vi "CRYConfigure Step.vi"(11 "Project Tree reference":refnum<vi>) -> (1 "Steps config.":bool[](array[boolean]))   [LabVIEW 2013]
uses:
  <vilib>/Utility/miscctls.llb/LVStringsAndValuesArrayTypeDef.ctl
  CRYProject Editor Global.vi
panel:
  in  "Unit":string caption="单位"
  in  "Comment":string caption="注解"
  in  "Name":string caption="名字"
  in  "Overwrite":u16(slide) caption="UseMLVal_Level_1"
  in  "Y unit":string
  in  "Y dB ref":dbl=1.0 format="%.1f"
  in  "Y prefix":string
  in  "Y data":u16(ring)=1 items=["dB", "Lin"]
  in  "btnUnit":bool caption="units"
  in  "Iterations":i32 caption="迭代"
  in  "Increment":dbl=1.0 caption="增量" min=1.0 step=1.0
  in  "Start":dbl caption="开始" format="%#_5g"
  in  "Load Test":bool
  in  "After":bool caption="后"
  in  "counts jump":i32(ring)=4 items=["激励"=1, "采集"=2, "分析"=3, "后处理"=4, "上下限"=5]
  in  "fail jump":i32(ring)=4 items=["激励"=1, "采集"=2, "分析"=3, "后处理"=4, "上下限"=5]
  in  "pass jump":i32(ring)=4 items=["激励"=1, "采集"=2, "分析"=3, "后处理"=4, "上下限"=5]
  in  "Jump on FAIL to":bool caption="失败时跳转"
  in  "Jump on PASS to":bool caption="通过时跳转"
  in  "Halt on PASS":bool caption="通过时停止"
  in  "Halt on FAIL":bool caption="失败时停止"
  in  "Default action for new steps":bool caption="默认动作为新步骤"
  out "Step Name":string
  in  "wait for confirmation?":bool caption="显示确认"
  in  "Cancel button":bool
  in  "OK button":bool
  # "..................."
  # "..................."
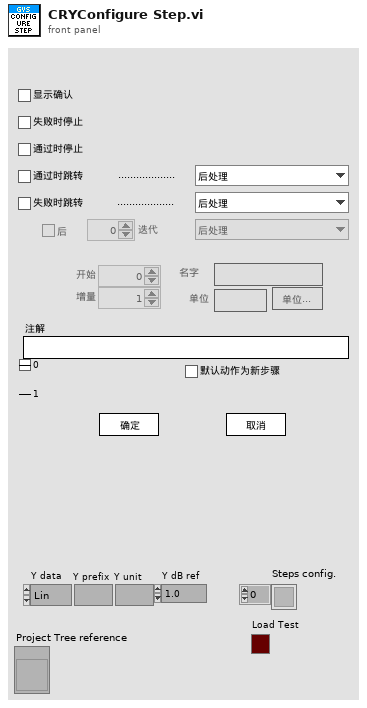
[diagram p1: front panel]
types:
  T1 = typedef "LVStringsAndValuesArrayTypeDef.ctl" = cluster{"String":string, "Value":ext}[]
  T2 = typedef "CRYTS.ctl" = cluster{"No.TS":u16, "TS File Path":path, "TS Name":string, "EditStepName":string, "Steps":T3[], "New State":bool, "Change State":bool, "Flattened CurveLib Data":string, "Document Data":string, "EditStepNo":u16, "Operator Start File":string, "Sequence Type":string, "Sequence Language":string}
  T3 = typedef "CRYStep.ctl" = cluster{"No.VI":i32, "Category":string, "StepName":string, "Seq setup flattened":string, "Comment":string, "Steps config.":bool[], "Jump config":i32[], "Start":dbl, "Increment":dbl, "Name":string, "Unit":string, "Y data":u16, "Y prefix":string, "Y dB ref":dbl, "Y unit":string, "Repeat State Array":cluster{"Start":dbl, "Increment":dbl, "Count":i32, "Num":i32}[]}
  T4 = typedef "CRYStart Cluster.ctl" = cluster{"SequenceName":string, "Preload Stimulus":bool, "CloseOpenedDisplay":bool, "ClearMeasuredData":bool, "UpdateDisplayDuringRun":bool, "DisplayForConfirmation":bool, "HaltOnFail":bool, "UseSameHardware":bool, "UseSameCalibration":bool}
  T5 = enum8{"Enabled", "Disabled", "Disabled and Grayed Out"}
  T6 = enum16{"Curves", "Values", "Results", "WFM", "All"}
  T7 = cluster{"SourceRowNum":i32, "SourceCount":i32, "TargetRowNum":i32, "bResult":bool, "EditRowNum":i32}
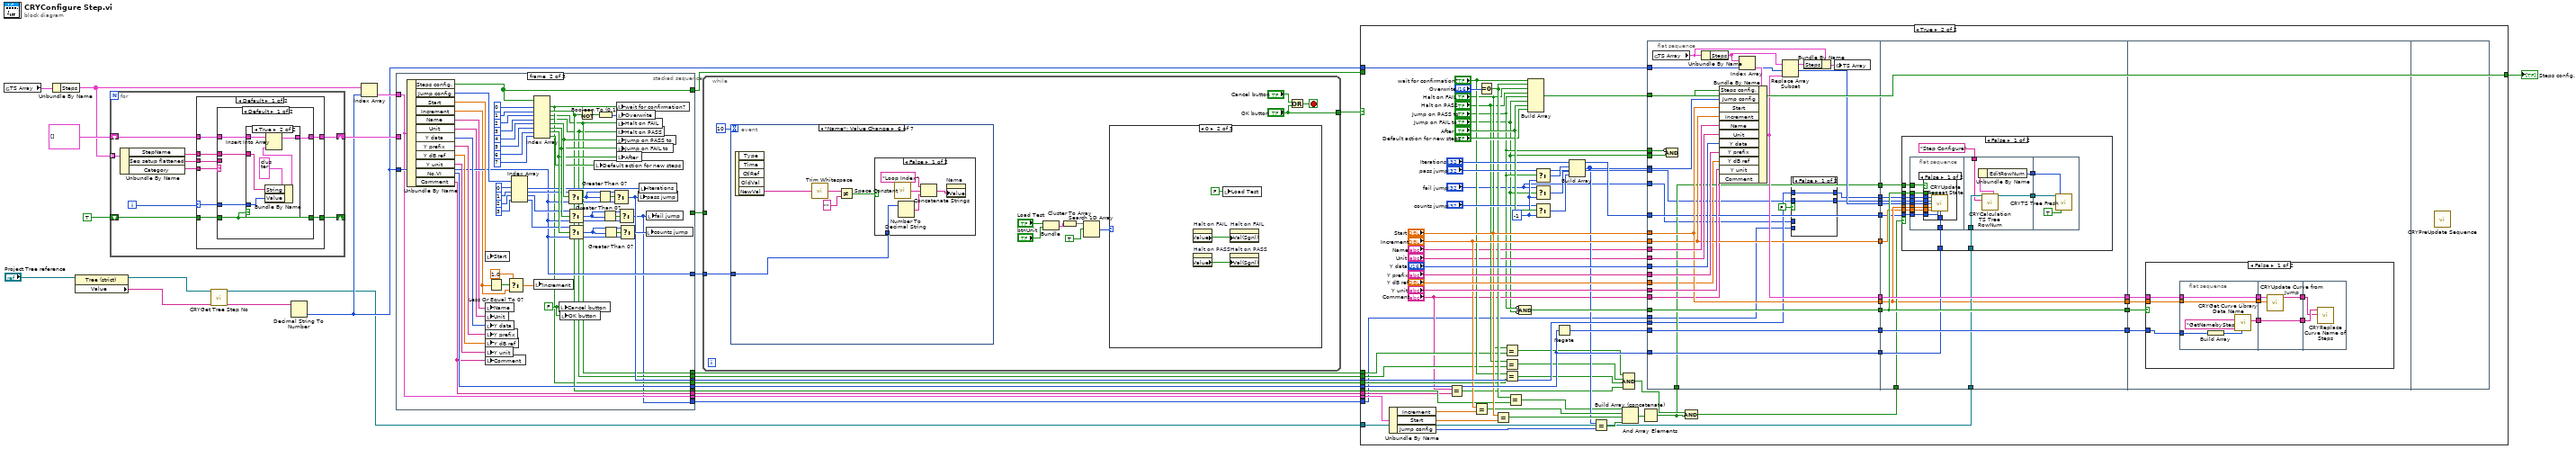
[diagram p0: block diagram]
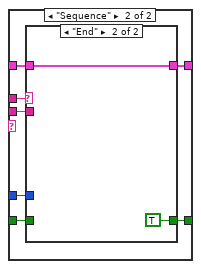
[diagram p3: hidden frame]
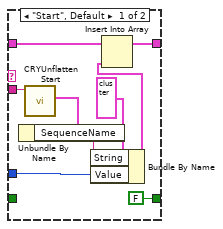
[diagram p4: hidden frame]
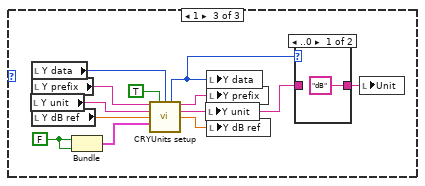
[diagram p7: hidden frame]
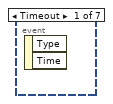
[diagram p9: hidden frame]
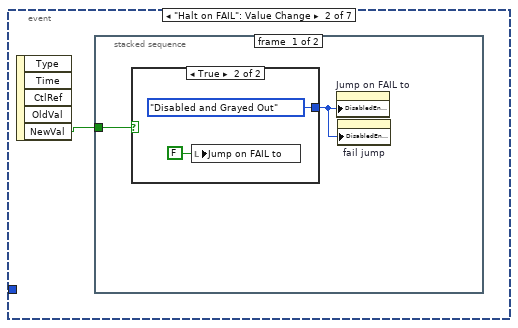
[diagram p10: hidden frame]
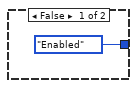
[diagram p11: hidden frame]
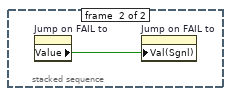
[diagram p12: hidden frame]
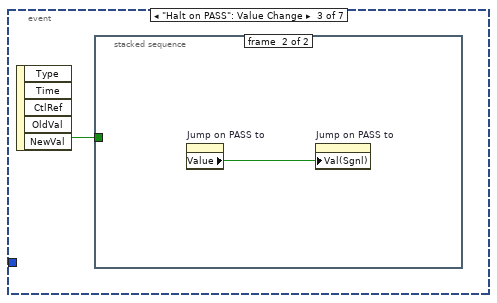
[diagram p13: hidden frame]
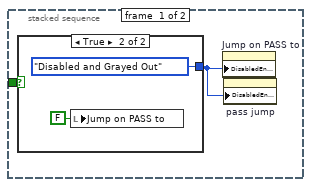
[diagram p14: hidden frame]
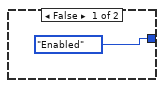
[diagram p15: hidden frame]
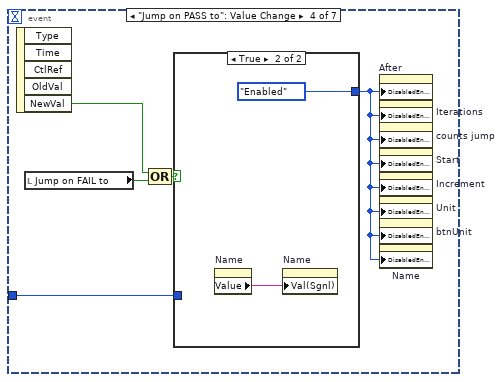
[diagram p16: hidden frame]
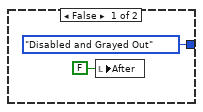
[diagram p17: hidden frame]
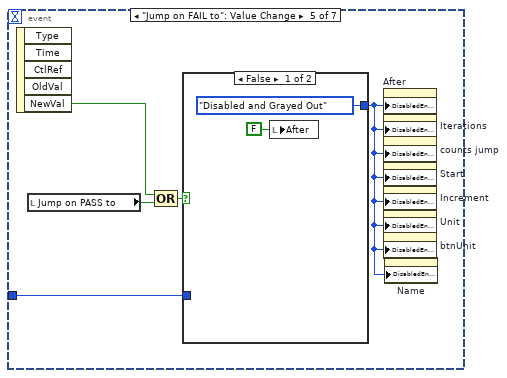
[diagram p18: hidden frame]
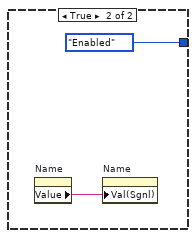
[diagram p19: hidden frame]
diagram:
  n1 = global read "CRYProject Editor Global.vi" "TS Array"() -> (w24:T2)
  n2 = Unbundle By Name(w24) -> ("Steps"=w16:T3[])
  n3 = property on="Property Node" class="Tree (strict)"(reference="Project Tree reference") -> (reference out=w7:refnum<vi>, "Value"=w6:string)  [unwired: 1 in, 1 out]
  n4 = for {
    tunnel: w16 -> [w34] mode=indexing
    shift-right: [w33] -> w18
    shift-left: T1 [] ("Strings And Values []") -> [w35]
    shift-right: [w30] -> _
    shift-left: TRUE ("Cancel button") -> [w31]
    i -> [w28]
    n5 = Unbundle By Name(w34) -> ("StepName"=w29:string, "Seq setup flattened"=w32:string, "Category"=w27:string)
    n6 = case shown="Default" w28 {
      selector: w28 -> [w39 _]
      tunnel: w35 -> [w42 w75]
      tunnel: [w40 w75] -> w33
      tunnel: w29 -> [w43 _]
      tunnel: w32 -> [w41 _]
      tunnel: w31 -> [w38 w74]
      tunnel: [w37 w74] -> w30
      tunnel: w27 -> [w36 _]
      frame Default {
        n7 = case shown="Default" w36 {
          tunnel: w43 -> [w45 w62]
          tunnel: w42 -> [w48 w61]
          tunnel: w41 -> [_ w60]
          tunnel: [w44 w59] -> w40
          tunnel: w39 -> [w46 w58]
          tunnel: w38 -> [w47 w57]
          tunnel: [w47 w56] -> w37
          frame Default {
            n8 = case shown="True" w47 {
              tunnel: w48 -> [w49 w55]
              tunnel: [w49 w54] -> w44
              tunnel: w45 -> [_ w52]
              tunnel: w46 -> [_ w51]
              frame False {
              }
              frame True {
                n9 = Bundle By Name(cluster=cluster{"String":string, "Value":ext} {"String"="", "Value"=0.0}, "String"=w52, "Value"=w51) -> (w50:cluster{"String":string, "Value":ext})
                n10 = Insert Into Array(array=w55, new element=w50) -> (w54:T1)  [unwired: 1 in]
              }
            }
          }
          frame "Sequence" {
            n11 = case shown="\"End\"" w62 {
              tunnel: w61 -> [w71 w73]
              tunnel: [w70 w73] -> w59
              tunnel: w60 -> [w69 _]
              tunnel: w58 -> [w64 _]
              tunnel: w57 -> [_ _]
              tunnel: [FALSE ("Cancel button") TRUE ("Cancel button")] -> w56
              frame "Start", Default {
                n12 = call "CRYUnflatten Start.vi"("Unflatten Sequence"=w69) -> ("Sequence Configure"=w68:T4)  [unwired: 8 in, 2 out]
                n13 = Unbundle By Name(w68) -> ("SequenceName"=w65:string)
                n14 = Bundle By Name(cluster=cluster{"String":string, "Value":ext} {"String"="", "Value"=0.0}, "String"=w65, "Value"=w64) -> (w63:cluster{"String":string, "Value":ext})
                n15 = Insert Into Array(array=w71, new element=w63) -> (w70:T1)  [unwired: 1 in]
              }
              frame "End" {
              }
            }
          }
        }
      }
      frame 0 {
      }
    }
  }
  n16 = call "CRYGet Tree Step No.vi"("SequenceTree"=w7, "Active Item Tag"=w6) -> ("reference out"=w5:refnum<vi>, "Active Cell String4"=w4:string)  [unwired: 12 in]
  n17 = Decimal String To Number(string=w4) -> (number=w13:i32)  [unwired: 2 in, 1 out]
  n18 = Index Array(array=w16, index=w13) -> (element=w15:T3)
  n19 = stacked-sequence {
    tunnel: w18 -> [w80 _ _]
    tunnel: w13 -> [_ w101 _]
    tunnel: w15 -> [w77 w93 _]
    tunnel: [_ w113 _] -> w23
    tunnel: [_ _ w134] -> w22
    tunnel: [_ w101 _] -> w21
    tunnel: [_ w107 _] -> w20
    tunnel: [_ w94 _] -> w12
    tunnel: [_ w93 _] -> w11
    tunnel: [_ w92 _] -> w10
    tunnel: [_ w87 _] -> w9
    tunnel: [_ w91 _] -> w8
    tunnel: [_ w90 _] -> w3
    tunnel: [_ w89 _] -> w2
    tunnel: [_ w85 _] -> w1
    frame #0 {
      n20 = Unbundle By Name(w77) -> ("StepName"=→"Step Name":string)
      n21 = Array Subset(array=w80, index=0) -> (w78:T1)  [unwired: 1 in]
      n22 = property on="pass jump" class="Ring (strict)"("StringsAndValues[]"=w78) -> ()  [unwired: 2 in, 2 out]
      n23 = property on="fail jump" class="Ring (strict)"("StringsAndValues[]"=w78) -> ()  [unwired: 2 in, 2 out]
      n24 = property on="counts jump" class="Ring (strict)"("StringsAndValues[]"=w78) -> ()  [unwired: 2 in, 2 out]
    }
    frame #1 {
      w131 = FALSE ("Cancel button")
      n25 = Unbundle By Name(w93) -> ("Steps config."=w113:bool[], "Jump config"=w114:i32[], "Start"=w112:dbl, "Increment"=w82:dbl, "Name"=w88:string, "Unit"=w86:string, "Y data"=w111:u16, "Y prefix"=w110:string, "Y dB ref"=w109:dbl, "Y unit"=w108:string, "No.VI"=w107:i32, "Comment"=w87:string)
      n26 = local write "Start"(w112) -> ()
      n27 = local write "Name"(w88) -> ()
      n28 = local write "Unit"(w86) -> ()
      n29 = local write "Y data"(w111) -> ()
      n30 = local write "Y prefix"(w110) -> ()
      n31 = local write "Y dB ref"(w109) -> ()
      n32 = local write "Y unit"(w108) -> ()
      n33 = local write "Comment"(w87) -> ()
      n34 = Less Or Equal To 0?(x=w82) -> (x <= 0?=w84:bool)
      n35 = Select(t=1.0, s=w84, f=w82) -> (s? t:f=w81:dbl)
      n36 = Index Array(array=w114, index #1=0 ("index"), index #2=1 ("index"), index #3=2 ("index"), index #4=3 ("index")) -> (element #1=w115:i32, element #2=w116:i32, element #3=w118:i32, element #4=w117:i32)
      n37 = local write "Increment"(w81) -> ()
      n38 = Index Array(array=w113, index #1=0 ("index"), index #2=1 ("index"), index #3=2 ("index"), index #4=3 ("index"), index #5=4 ("index"), index #6=5 ("index"), index #7=6 ("index"), index #8=7 ("index")) -> (element #1=w91:bool, element #2=w92:bool, element #3=w90:bool, element #4=w89:bool, element #5=w121:bool, element #6=w120:bool, element #7=w119:bool, element #8=w95:bool)
      n39 = local write "Cancel button"(w131) -> ()
      n40 = local write "OK button"(w131) -> ()
      n41 = Select(t=w116, s=w121, f=w101) -> (s? t:f=w105:i32)
      n42 = Select(t=w118, s=w120, f=w101) -> (s? t:f=w103:i32)
      n43 = Select(t=w117, s=w119, f=w101) -> (s? t:f=w100:i32)
      n44 = Not(x=w92) -> (.not. x?=w97:bool)
      n45 = local write "Default action for new steps"(w95) -> ()
      n46 = Greater Than 0?(x=w105) -> (x > 0?=w106:bool)
      n47 = Boolean To (0,1)(Boolean=w97) -> (0, 1=w98:i16)
      n48 = Greater Than 0?(x=w103) -> (x > 0?=w104:bool)
      n49 = Greater Than 0?(x=w100) -> (x > 0?=w102:bool)
      n50 = Select(t=w105, s=w106, f=w101) -> (s? t:f=w94:i32)
      n51 = local write "wait for confirmation?"(w91) -> ()
      n52 = local write "Overwrite"(w98) -> ()
      n53 = local write "Halt on FAIL"(w90) -> ()
      n54 = local write "Halt on PASS"(w89) -> ()
      n55 = local write "Jump on PASS to"(w121) -> ()
      n56 = local write "Jump on FAIL to"(w120) -> ()
      n57 = local write "After"(w119) -> ()
      n58 = Select(t=w103, s=w104, f=w101) -> (s? t:f=w85:i32)
      n59 = Select(t=w100, s=w102, f=w101) -> (s? t:f=w99:i32)
      n60 = local write "pass jump"(w94) -> ()
      n61 = local write "Iterations"(w115) -> ()
      n62 = local write "counts jump"(w99) -> ()
      n63 = local write "fail jump"(w85) -> ()
    }
    frame #2 {
      w134 = TRUE ("Load Test")
      n64 = control-ref of="This VI"() -> (w135:refnum<vi>)
      n65 = call "CRYGet Window Title Message.vi"("No"=6, "Kind"="Project") -> ("Multibyte String"=w136:string)  [unwired: 4 in, 5 out]
      n66 = call "CRYConfigure Step Front Panel.vi"("Vi Ref"=w135) -> ()  [unwired: 11 in]
      n67 = property class="VI"(reference=w135, "Front Panel.Title"=w136) -> ()  [unwired: 1 in, 2 out]
      n68 = local write "Load Test"(w134) -> ()
    }
  }
  n69 = while {
    tunnel: ["OK button"] -> w26
    tunnel: w22 -> [_]
    tunnel: w21 -> [w139]
    stop <- w149 stop-if-true
    n70 = event shown="[5] \"Name\": Value Change" {
      selector: _ -> [_ _ _ _ _ _ _]
      dyn-events: _ -> [_ _ _ _ _ _ _]
      timeout: 10 -> [_ _ _ _ _ _ _]
      tunnel: w139 -> [_ _ _ w182 w191 w200 _]
      event Timeout {
        n71 = event-data() -> ()  [unwired: 1 in, 2 out]
      }
      event "Halt on FAIL": Value Change {
        n72 = event-data() -> ("NewVal"=w167:bool)  [unwired: 1 in, 4 out]
        n73 = stacked-sequence {
          tunnel: w167 -> [w168 _]
          frame #0 {
            n74 = case shown="True" w168 {
              tunnel: [T5."Enabled" ("Disabled") T5."Disabled and Grayed Out" ("Disabled")] -> w169
              frame False {
              }
              frame True {
                n75 = local write "Jump on FAIL to"(FALSE ("Jump on FAIL to")) -> ()
              }
            }
            n76 = property on="Jump on FAIL to" class="Bool (strict)"("DisabledEnum"=w169) -> ()  [unwired: 2 in, 2 out]
            n77 = property on="fail jump" class="Ring (strict)"("DisabledEnum"=w169) -> ()  [unwired: 2 in, 2 out]
          }
          frame #1 {
            n78 = property on="Jump on FAIL to" class="Bool (strict)"() -> ("Value"=w173:bool)  [unwired: 2 in, 2 out]
            n79 = property on="Jump on FAIL to" class="Bool (strict)"("Val(Sgnl)"=w173) -> ()  [unwired: 2 in, 2 out]
          }
        }
      }
      event "Halt on PASS": Value Change {
        n80 = event-data() -> ("NewVal"=w174:bool)  [unwired: 1 in, 4 out]
        n81 = stacked-sequence {
          tunnel: w174 -> [w175 _]
          frame #0 {
            n82 = case shown="True" w175 {
              tunnel: [T5."Enabled" ("Disabled") T5."Disabled and Grayed Out" ("Disabled")] -> w176
              frame False {
              }
              frame True {
                n83 = local write "Jump on PASS to"(FALSE ("Jump on PASS to")) -> ()
              }
            }
            n84 = property on="Jump on PASS to" class="Bool (strict)"("DisabledEnum"=w176) -> ()  [unwired: 2 in, 2 out]
            n85 = property on="pass jump" class="Ring (strict)"("DisabledEnum"=w176) -> ()  [unwired: 2 in, 2 out]
          }
          frame #1 {
            n86 = property on="Jump on PASS to" class="Bool (strict)"() -> ("Value"=w180:bool)  [unwired: 2 in, 2 out]
            n87 = property on="Jump on PASS to" class="Bool (strict)"("Val(Sgnl)"=w180) -> ()  [unwired: 2 in, 2 out]
          }
        }
      }
      event "Jump on PASS to": Value Change {
        n88 = event-data() -> ("NewVal"=w183:bool)  [unwired: 1 in, 4 out]
        n89 = local read "Jump on FAIL to"() -> (w185:bool)
        n90 = Compound Arithmetic op=OR(w183, w185) -> (w184:bool)
        n91 = case shown="True" w184 {
          tunnel: [T5."Disabled and Grayed Out" ("Disabled") T5."Enabled" ("Disabled")] -> w181
          tunnel: w182 -> [_ _]
          frame False {
            n92 = local write "After"(FALSE ("After")) -> ()
          }
          frame True {
            n93 = property on="Name" class="Str"() -> ("Value"=w188:string)  [unwired: 2 in, 2 out]
            n94 = property on="Name" class="Str"("Val(Sgnl)"=w188) -> ()  [unwired: 2 in, 2 out]
          }
        }
        n95 = property on="After" class="Bool (strict)"("DisabledEnum"=w181) -> ()  [unwired: 2 in, 2 out]
        n96 = property on="Iterations" class="DigNum (strict)"("DisabledEnum"=w181) -> ()  [unwired: 2 in, 2 out]
        n97 = property on="counts jump" class="Ring (strict)"("DisabledEnum"=w181) -> ()  [unwired: 2 in, 2 out]
        n98 = property on="Start" class="DigNum (strict)"("DisabledEnum"=w181) -> ()  [unwired: 2 in, 2 out]
        n99 = property on="Increment" class="DigNum (strict)"("DisabledEnum"=w181) -> ()  [unwired: 2 in, 2 out]
        n100 = property on="Unit" class="Str"("DisabledEnum"=w181) -> ()  [unwired: 2 in, 2 out]
        n101 = property on="btnUnit" class="Bool"("DisabledEnum"=w181) -> ()  [unwired: 2 in, 2 out]
        n102 = property on="Name" class="Str"("DisabledEnum"=w181) -> ()  [unwired: 2 in, 2 out]
      }
      event "Jump on FAIL to": Value Change {
        n103 = event-data() -> ("NewVal"=w193:bool)  [unwired: 1 in, 4 out]
        n104 = local read "Jump on PASS to"() -> (w192:bool)
        n105 = Compound Arithmetic op=OR(w193, w192) -> (w194:bool)
        n106 = case shown="False" w194 {
          tunnel: [T5."Disabled and Grayed Out" ("Disabled") T5."Enabled" ("Disabled")] -> w190
          tunnel: w191 -> [_ _]
          frame False {
            n107 = local write "After"(FALSE ("After")) -> ()
          }
          frame True {
            n108 = property on="Name" class="Str"() -> ("Value"=w197:string)  [unwired: 2 in, 2 out]
            n109 = property on="Name" class="Str"("Val(Sgnl)"=w197) -> ()  [unwired: 2 in, 2 out]
          }
        }
        n110 = property on="After" class="Bool (strict)"("DisabledEnum"=w190) -> ()  [unwired: 2 in, 2 out]
        n111 = property on="Iterations" class="DigNum (strict)"("DisabledEnum"=w190) -> ()  [unwired: 2 in, 2 out]
        n112 = property on="counts jump" class="Ring (strict)"("DisabledEnum"=w190) -> ()  [unwired: 2 in, 2 out]
        n113 = property on="Start" class="DigNum (strict)"("DisabledEnum"=w190) -> ()  [unwired: 2 in, 2 out]
        n114 = property on="Increment" class="DigNum (strict)"("DisabledEnum"=w190) -> ()  [unwired: 2 in, 2 out]
        n115 = property on="Unit" class="Str"("DisabledEnum"=w190) -> ()  [unwired: 2 in, 2 out]
        n116 = property on="btnUnit" class="Bool"("DisabledEnum"=w190) -> ()  [unwired: 2 in, 2 out]
        n117 = property on="Name" class="Str"("DisabledEnum"=w190) -> ()  [unwired: 2 in, 2 out]
      }
      event "Name": Value Change {
        n118 = event-data() -> ("NewVal"=w199:string)  [unwired: 1 in, 4 out]
        n119 = call <vilib>:"Trim Whitespace.vi"("string"=w199) -> ("trimmed string"=w203:string)  [unwired: 1 in]
        n120 = Not Equal?(x=w203, y="") -> (x != y?=w201:bool)
        n121 = case shown="False" w201 {
          tunnel: w200 -> [w207 _]
          frame False {
            n122 = call <vilib>:"Space Constant.vi"() -> ("String"=w204:string)
            n123 = Number To Decimal String(number=w207) -> (decimal integer string=w208:string)  [unwired: 1 in]
            n124 = Concatenate Strings("Loop Index" ("Name"), w204, w208) -> (w206:string)
            n125 = property on="Name" class="Str"("Value"=w206) -> ()  [unwired: 2 in, 2 out]
          }
          frame True {
          }
        }
      }
      event Panel Close? {
        w209 = TRUE ("Discard?")
        n126 = event-data() -> ()  [unwired: 1 in, 3 out]
        n127 = local write "Cancel button"(w209) -> ()
        n128 = event-data("Discard?"=w209) -> ()  [unwired: 1 in, 1 out]
      }
    }
    n129 = Bundle("Load Test"="Load Test", "btnUnit"="btnUnit") -> (w145:cluster{"Load Test":bool, "btnUnit":bool})  [unwired: 1 out]
    n130 = Cluster To Array(cluster=w145) -> (array=w144:bool[])
    n131 = Search 1D Array(1D array=w144, element=TRUE) -> (index of element=w141:i32)  [unwired: 1 out]
    n132 = case shown="0" w141 {
      frame Default {
      }
      frame 0 {
        n133 = property on="Halt on FAIL" class="Bool (strict)"() -> ("Value"=w150:bool)  [unwired: 2 in, 2 out]
        n134 = property on="Halt on PASS" class="Bool (strict)"() -> ("Value"=w151:bool)  [unwired: 2 in, 2 out]
        n135 = local write "Load Test"(FALSE ("Load Test")) -> ()
        n136 = property on="Halt on FAIL" class="Bool (strict)"("Val(Sgnl)"=w150) -> ()  [unwired: 2 in, 2 out]
        n137 = property on="Halt on PASS" class="Bool (strict)"("Val(Sgnl)"=w151) -> ()  [unwired: 2 in, 2 out]
      }
      frame 1 {
        w163 = FALSE
        n138 = local read "Y unit"() -> (w159:string)
        n139 = local read "Y data"() -> (w161:u16)
        n140 = local read "Y prefix"() -> (w160:string)
        n141 = local read "Y dB ref"() -> (w158:dbl)
        n142 = Bundle(w163, w163) -> (w164:cluster{bool, bool})  [unwired: 1 out]
        n143 = call "CRYUnits setup.vi"("unit prefix"=w160, "Scale visible?"=TRUE, "dB/Lin"=w161, "Unit:"=w159, "dB ref:"=w158, "Custom unit settings"=w164) -> ("New Scale"=w155:u16, "New unit prefix Lin"=w157:string, "New unit Lin"=w154:string, "New dB ref"=w156:dbl)  [unwired: 2 in, 4 out]
        n144 = local write "Y unit"(w154) -> ()
        n145 = local write "Y data"(w155) -> ()
        n146 = local write "Y prefix"(w157) -> ()
        n147 = local write "Y dB ref"(w156) -> ()
        n148 = case shown="..0" w155 {
          tunnel: ["dB" w166] -> w153
          tunnel: w154 -> [_ w166]
          frame ..0 {
          }
          frame 1.. {
          }
        }
        n149 = local write "Unit"(w153) -> ()
      }
    }
    n150 = Or(x="Cancel button", y="OK button") -> (x .or. y?=w149:bool)
  }
  n151 = case shown="True" w26 {
    tunnel: w23 -> [w210 _]
    tunnel: [w210 w281] -> w25
    tunnel: w13 -> [_ w267]
    tunnel: w20 -> [_ w265]
    tunnel: w12 -> [_ w266]
    tunnel: w11 -> [_ w264]
    tunnel: w10 -> [_ w249]
    tunnel: w5 -> [_ w239]
    tunnel: w9 -> [_ w232]
    tunnel: w8 -> [_ w230]
    tunnel: w3 -> [_ w223]
    tunnel: w2 -> [_ w222]
    tunnel: w1 -> [_ w211]
    frame False {
    }
    frame True {
      w277 = -1 ("f")
      n152 = Unbundle By Name(w264) -> ("Increment"=w263:dbl, "Start"=w260:dbl, "Jump config"=w252:i32[])
      n153 = Equal?(x="Comment", y=w232) -> (x = y?=w228:bool)
      n154 = Equal?(x="Increment", y=w263) -> (x = y?=w256:bool)
      n155 = Equal To 0?(x="Overwrite") -> (x = 0?=w250:bool)
      n156 = Equal?(x="Start", y=w260) -> (x = y?=w255:bool)
      n157 = Equal?(x="Halt on FAIL", y=w223) -> (x = y?=w221:bool)
      n158 = Equal?(x="Halt on PASS", y=w222) -> (x = y?=w220:bool)
      n159 = Equal?(x="wait for confirmation?", y=w230) -> (x = y?=w229:bool)
      n160 = Equal?(x=w250, y=w249) -> (x = y?=w248:bool)
      n161 = Compound Arithmetic op=AND(invert "Jump on PASS to", invert "Jump on FAIL to") -> (w271:bool)
      n162 = Build Array("wait for confirmation?", w250, "Halt on FAIL", "Halt on PASS", "Jump on PASS to", "Jump on FAIL to", "After", "Default action for new steps") -> (w281:bool[])
      n163 = Select(t="pass jump", s="Jump on PASS to", f=w277) -> (s? t:f=w280:i32)
      n164 = Select(t="fail jump", s="Jump on FAIL to", f=w277) -> (s? t:f=w279:i32)
      n165 = Select(t="counts jump", s="After", f=w277) -> (s? t:f=w276:i32)
      n166 = Negate(x=w265) -> (-x=w270:i32)
      n167 = Build Array("Iterations", w280, w279, w276) -> (w253:i32[])
      n168 = Equal?(x=w253, y=w252) -> (x = y?=w251:bool[])
      n169 = Build Array (concatenate)(w248, w256, w255, w251) -> (w254:bool[])
      n170 = Compound Arithmetic op=AND(w221, w220, w229, w228) -> (w227:bool)
      n171 = And Array Elements(Boolean array=w254) -> (logical AND=w218:bool)
      n172 = flat-sequence {
        tunnel: [w301] -> w247
        tunnel: [w300] -> w245
        tunnel: [w299] -> w243
        tunnel: [w298] -> w241
        tunnel: [w297] -> w238
        tunnel: [w296] -> w237
        tunnel: [w287] -> w236
        tunnel: [w285] -> w235
        tunnel: [w295] -> w234
        tunnel: [w294] -> w233
        tunnel: w281 -> [w312]
        tunnel: w253 -> [w310]
        tunnel: "Increment" -> [w296]
        tunnel: "Name" -> [w309]
        tunnel: "Unit" -> [w308]
        tunnel: "Y data" -> [w307]
        tunnel: "Y prefix" -> [w306]
        tunnel: "Y dB ref" -> [w291]
        tunnel: "Y unit" -> [w305]
        tunnel: w271 -> [w299]
        tunnel: "Start" -> [w300]
        tunnel: w270 -> [w298]
        tunnel: w267 -> [w295]
        tunnel: w265 -> [w297]
        tunnel: w266 -> [w288]
        tunnel: "pass jump" -> [w286]
        tunnel: "Iterations" -> [w294]
        tunnel: "Comment" -> [w293]
        tunnel: [w292] -> w219
        tunnel: w218 -> [w292]
        tunnel: "Jump on PASS to" -> [w290]
        tunnel: "Jump on FAIL to" -> [w289]
        tunnel: "fail jump" -> [w284]
        tunnel: w211 -> [w283]
        tunnel: w247 -> [w330]
        tunnel: [w330] -> w246
        tunnel: w245 -> [w324]
        tunnel: [w324] -> w244
        tunnel: w243 -> [w328]
        tunnel: [w328] -> w242
        tunnel: w241 -> [w329]
        tunnel: [w329] -> w240
        tunnel: w239 -> [w327]
        tunnel: w238 -> [w326]
        tunnel: w226 -> [w325]
        tunnel: w237 -> [w323]
        tunnel: w236 -> [w322]
        tunnel: w235 -> [w321]
        tunnel: w234 -> [w320]
        tunnel: w233 -> [w319]
        tunnel: w219 -> [w318]
        tunnel: w246 -> [w372]
        tunnel: w244 -> [w371]
        tunnel: w242 -> [w370]
        tunnel: w240 -> [w369]
        frame #0 {
          n173 = global read "CRYProject Editor Global.vi" "TS Array"() -> (w302:T2)
          n174 = Compound Arithmetic op=AND(invert w290, w289) -> ()  [unwired: 1 out]
          n175 = Unbundle By Name(w302) -> ("Steps"=w303:T3[])
          n176 = Index Array(array=w303, index=w295) -> (element=w304:T3)
          n177 = Bundle By Name(cluster=w304, "Steps config."=w312, "Jump config"=w310, "Start"=w300, "Increment"=w296, "Name"=w309, "Unit"=w308, "Y data"=w307, "Y prefix"=w306, "Y dB ref"=w291, "Y unit"=w305, "Comment"=w293) -> (w301:T3)
          n178 = Replace Array Subset(array=w303, new element=w301, index=w295) -> (w313:T3[])
          n179 = case shown="False" FALSE {
            tunnel: w288 -> [w315 _]
            tunnel: [w315 w316] -> w287
            tunnel: w286 -> [w314 _]
            tunnel: [w314 w317] -> w285
            tunnel: w284 -> [_ w317]
            tunnel: w283 -> [_ w316]
            frame False {
            }
            frame True {
            }
          }
          n180 = Bundle By Name(cluster=w302, "Steps"=w313) -> (w311:T2)
          n181 = global write "CRYProject Editor Global.vi" "TS Array"(w311) -> ()
        }
        frame #1 {
          n182 = case shown="False" w325 {
            tunnel: w319 -> [w343 _]
            tunnel: w328 -> [w342 _]
            tunnel: w320 -> [w341 _]
            tunnel: w324 -> [w340 _]
            tunnel: w323 -> [w339 _]
            tunnel: w322 -> [w338 _]
            tunnel: w321 -> [w337 _]
            tunnel: w326 -> [w336 _]
            tunnel: w327 -> [w335 _]
            tunnel: w318 -> [w331 _]
            frame False {
              n183 = flat-sequence {
                tunnel: w343 -> [w352]
                tunnel: w342 -> [w351]
                tunnel: w341 -> [w350]
                tunnel: w340 -> [w349]
                tunnel: w339 -> [w348]
                tunnel: w338 -> [w347]
                tunnel: w337 -> [w346]
                tunnel: w336 -> [w345]
                tunnel: w331 -> [w344]
                tunnel: w335 -> [w365]
                tunnel: [w364] -> w334
                tunnel: "Step Configure" ("sOption") -> [w363]
                tunnel: [w361] -> w332
                tunnel: w334 -> [w367]
                tunnel: w332 -> [w366]
                frame #0 {
                  n184 = case shown="False" w344 {
                    tunnel: w352 -> [w360 _]
                    tunnel: w351 -> [w359 _]
                    tunnel: w350 -> [w358 _]
                    tunnel: w349 -> [w357 _]
                    tunnel: w348 -> [w356 _]
                    tunnel: w347 -> [w355 _]
                    tunnel: w346 -> [w354 _]
                    tunnel: w345 -> [w353 _]
                    frame False {
                      n185 = call "CRYUpdate Repeat State.vi"("destination Index1"=w355, "fOption"=w359, "destination Index2"=w354, "My Index"=w358, "Start"=w357, "Increment"=w356, "Count"=w360, "VI No"=w353) -> ()  [unwired: 7 in, 1 out]
                    }
                    frame True {
                    }
                  }
                }
                frame #1 {
                  n186 = call "CRYCalculation TS Tree RowNum.vi"("Tree Task SequenceIn"=w365, "sOption"=w363) -> ("DispInfo Cluster Out"=w362:T7, "Tree Task Sequence Out"=w364:refnum<vi>)  [unwired: 7 in, 5 out]
                  n187 = Unbundle By Name(w362) -> ("EditRowNum"=w361:i32)
                }
                frame #2 {
                  n188 = call "CRYTS Tree Fresh.vi"("SequenceTree"=w367, "Edit Index"=w366, "Is Refresh?"=TRUE) -> ()  [unwired: 12 in, 1 out]
                }
              }
            }
            frame True {
            }
          }
        }
        frame #2 {
          n189 = case shown="False" w370 {
            tunnel: w369 -> [w379 w394]
            tunnel: w372 -> [w378 _]
            tunnel: w371 -> [w380 _]
            frame False {
              n190 = flat-sequence {
                tunnel: w380 -> [w385]
                tunnel: w378 -> [w386]
                tunnel: [w386] -> w377
                tunnel: [w385] -> w376
                tunnel: w379 -> [w384]
                tunnel: [w383] -> w375
                tunnel: w377 -> [w390]
                tunnel: w376 -> [w389]
                tunnel: [w388] -> w374
                tunnel: w375 -> [w388]
                tunnel: [w387] -> w373
                tunnel: w374 -> [w392]
                tunnel: w373 -> [w391]
                frame #0 {
                  n191 = Build Array(w384) -> (w382:i32[])
                  n192 = call "CRYGet Curve Library Data Name.vi"("nData"=w382, "sAction"="GetNamebyStep" ("sOption")) -> ("sNames"=w383:string[])  [unwired: 6 in, 3 out]
                }
                frame #1 {
                  n193 = call "CRYUpdate Curve from Jump.vi"("Y Value"=w389, "Step Configure"=w390) -> ("Inserted Names Out"=w387:string[])  [unwired: 9 in]
                }
                frame #2 {
                  n194 = call "CRYReplace Curve Name of Steps.vi"("New Name"=w391, "Old Name"=w392) -> ()  [unwired: 9 in, 1 out]
                }
              }
            }
            frame True {
              n195 = Build Array(w394) -> (w393:i32[])
              n196 = call "CRYDelete Complete From Step.vi"("Step No."=w393, "Type In"=T6."Values") -> ()  [unwired: 10 out]
            }
          }
        }
        frame #3 {
          n197 = call "CRYPreUpdate Sequence.vi"() -> ()  [unwired: 16 in]
        }
      }
      n198 = Compound Arithmetic op=AND(w227, w218) -> (w226:bool)
    }
  }
  "Steps config." <- w25
